vi "Erase Metrics.vi"(8 "error in (no error)":errorcluster, 11 "Default Collector in":refnum<class "Default Collector.lvclass">) -> (0 "error out":errorcluster, 3 "Default Collector out":refnum<class "Default Collector.lvclass">)   [LabVIEW 2020, in "Collector.lvlib" / "Default Collector.lvclass"]
uses:
  Default Collector.lvclass
  Default Collector.lvclass/Default Collector.ctl
  metrics/metric/Metric.lvclass
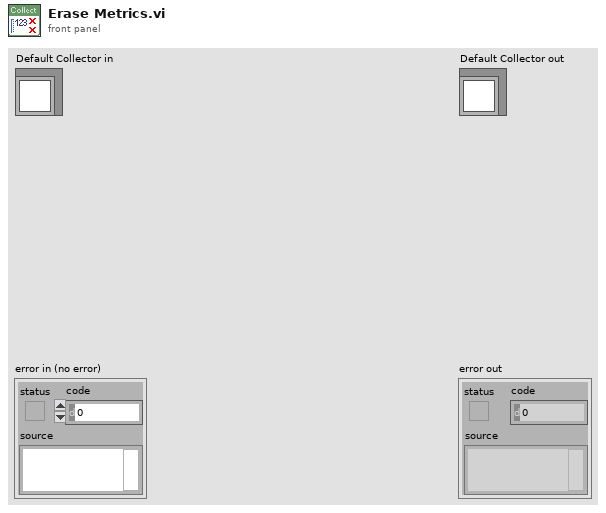
[diagram p1: front panel]
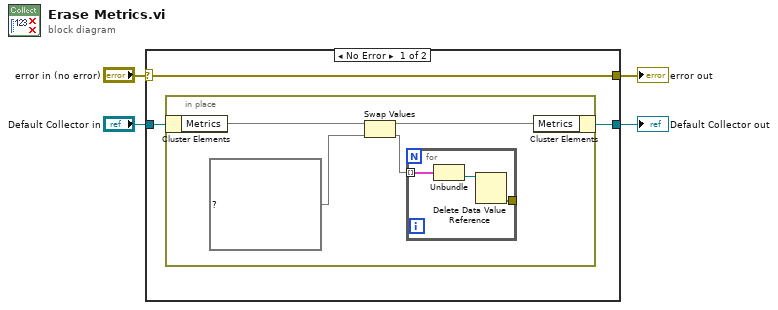
[diagram p0: block diagram]
diagram:
  n1 = case shown="No Error" "error in (no error)" {
    selector: "error in (no error)" -> [w7 w16]
    tunnel: [w7 w16] -> w3
    tunnel: [w5 w15] -> w1
    tunnel: "Default Collector in" -> [w6 w15]
    frame No Error {
      n2 = in-place {
        n3 = in-place-cluster #1(w6) -> ("Metrics"=w11:map{string, refnum<data-value>})
        n4 = Swap Values(12:w11, 14:map{string, refnum<data-value>} {} ("Metrics")) -> (1:w9:map{string, refnum<data-value>}, 3:w8:map{string, refnum<data-value>})  [unwired: 1 in]
        n5 = for {
          tunnel: w8 -> [w14] mode=indexing
          tunnel: [w12] -> _
          n6 = Unbundle(w14) -> ("Metric"=w13:refnum<data-value>)  [unwired: 1 out]
          n7 = Delete Data Value Reference(data value reference=w13) -> (error out=w12:errorcluster)  [unwired: 1 in, 1 out]
        }
        n8 = in-place-cluster #1("Metrics"=w9) -> (w5:refnum<class "Default Collector.lvclass">)
      }
    }
    frame Error {
    }
  }
  "error out" <- w3
  "Default Collector out" <- w1
